vi "Configure System Prompt.vi"(8 "error in (no error)":errorcluster, 10 "System Prompt State (F: Disable)":bool, 11 "VISA resource name":refnum<visa-resource-name>) -> (0 "error out":errorcluster, 3 "VISA resource name out":refnum<visa-resource-name>)   [LabVIEW 2018, in "XP Power PLS600.lvlib"]
doc: "Enables (On) or disables (Off) the SCPI prompt. The prompt is the text string “>>”."
uses:
  XP Power PLS600.lvlib
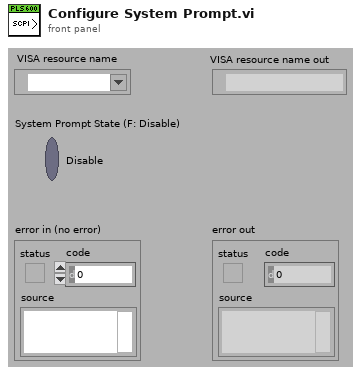
[diagram p1: front panel]
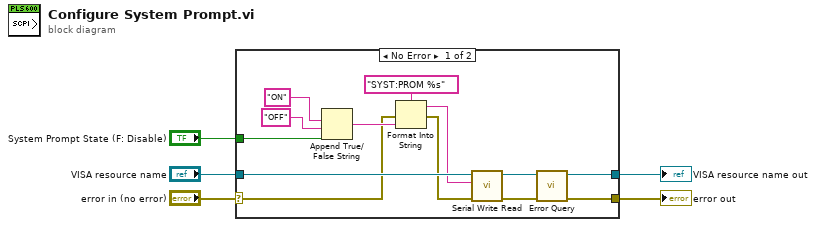
[diagram p0: block diagram]
diagram:
  n1 = case shown="No Error" "error in (no error)" {
    selector: "error in (no error)" -> [w6 w20]
    tunnel: "System Prompt State (F: Disable)" -> [w18 _]
    tunnel: [w17 w19] -> w4
    tunnel: [w16 w20] -> w3
    tunnel: "VISA resource name" -> [w13 w19]
    frame No Error {
      n2 = Append True/False String(1:w18, 2:"OFF", 3:"ON") -> (0:w9:string)  [unwired: 1 in]
      n3 = Format Into String(format string="SYST:PROM %s" ("Command to Send"), error in=w6, w9) -> (resulting string=w8:string, error out=w7:errorcluster)  [unwired: 1 in]
      n4 = call "Serial Write Read.vi"("error in (no error)"=w7, "Write Buffer"=w8, "VISA resource name"=w13) -> ("error out"=w11:errorcluster, "VISA resource name out"=w12:refnum<visa-resource-name>)  [unwired: 6 in, 1 out]
      n5 = call "Error Query.vi"("error in (no error)"=w11, "VISA resource name"=w12) -> ("error out"=w16:errorcluster, "VISA resource name out"=w17:refnum<visa-resource-name>)  [unwired: 6 in, 2 out]
    }
    frame Error {
    }
  }
  "VISA resource name out" <- w4
  "error out" <- w3
